vi "stereo_cam_aquisition.vi"() -> ()   [LabVIEW 2015]
uses:
  <vilib>/userdefined/High Color/IMAQdx.ctl
  <vilib>/vision/driver/IMAQdx.llb/IMAQdx Acquisition Mode.ctl
  <vilib>/vision/driver/NI_Vision_Acquisition_Software.lvlib
  <vilib>/Analysis/NI_AALBase.lvlib
panel:
  in  "error in":errorcluster
  in  "stop":bool
  in  "bubnum #2":string
  in  "bubnum #1":string
  out "Absolute Difference in Entropy 2":dbl(graph)
  out "Absolute Difference in Entropy":dbl(graph)
  out "Camera Triggered":bool
  in  "Entropy Threshold":dbl
  out "Camera Image 2":T1(plugin-control)
  out "Buffer #2":u32
  out "Camera Image 1":T1(plugin-control)
  out "Buffer #1":u32
  in  "IMAQdx Session 2":T2
  in  "IMAQdx Session 1":T2
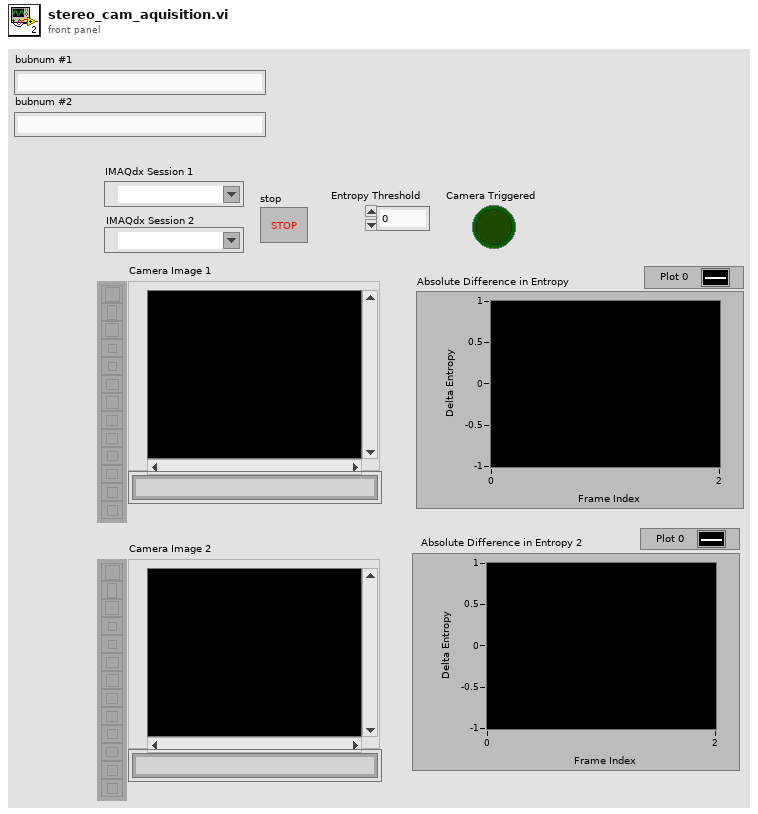
[diagram p1: front panel]
types:
  T1 = typedef "IMAQ Image.ctl" = refnum<image>
  T2 = typedef "IMAQdx.ctl" = refnum<k21>
  T3 = typedef "NI_Vision_Acquisition_Software.lvlib/IMAQdx Acquisition Mode.ctl" = enum32{"One Shot", "Continuous"}
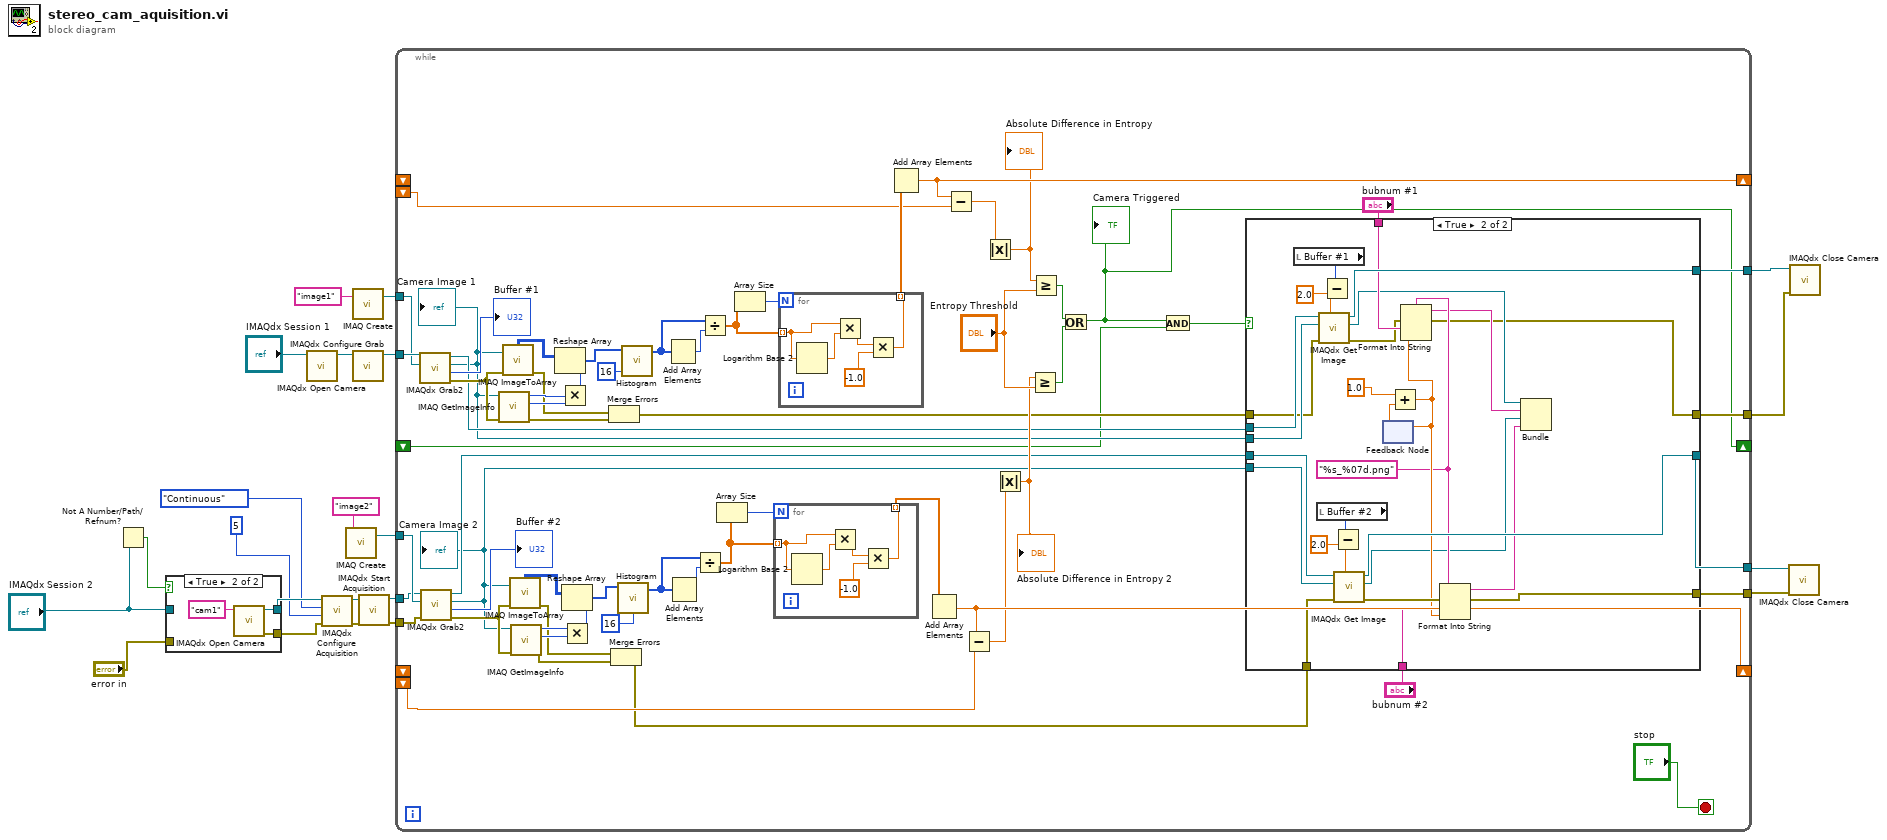
[diagram p0: block diagram]
diagram:
  n1 = Not A Number/Path/Refnum?(number/path/refnum="IMAQdx Session 2") -> (NaN/Path/Refnum?=w6:bool)
  n2 = case shown="True" w6 {
    tunnel: [w24 w27] -> w9
    tunnel: "IMAQdx Session 2" -> [w24 _]
    tunnel: [w23 w26] -> w10
    tunnel: "error in" -> [w23 _]
    frame False {
    }
    frame True {
      n3 = call <vilib>:"IMAQdx Open Camera.vi"("Session In"="cam1") -> ("error out"=w26:errorcluster, "Session Out"=w27:T2)  [unwired: 9 in]
    }
  }
  n4 = call <vilib>:"IMAQdx Open Camera.vi"("Session In"="IMAQdx Session 1") -> ("Session Out"=w22:T2)  [unwired: 9 in, 1 out]
  n5 = call <vilib>:"IMAQdx Configure Acquisition.vi"("error in"=w10, "Number of Buffers"=u32 5, "Continuous?"=IMAQdx_Acquisition_Mode."Continuous", "Session In"=w9) -> ("error out"=w4:errorcluster, "Session Out"=w3:T2)  [unwired: 6 in]
  n6 = call "IMAQ Create"("Image Name"="image2") -> ("New Image"=w18:T1)  [unwired: 4 in, 1 out]
  n7 = call "IMAQ Create"("Image Name"="image1") -> ("New Image"=w16:T1)  [unwired: 4 in, 1 out]
  n8 = call <vilib>:"IMAQdx Configure Grab.vi"("Session In"=w22) -> ("Session Out"=w17:T2)  [unwired: 9 in, 1 out]
  n9 = call <vilib>:"IMAQdx Start Acquisition.vi"("error in"=w4, "Session In"=w3) -> ("error out"=w1:errorcluster, "Session Out"=w2:T2)  [unwired: 8 in]
  n10 = while {
    tunnel: w18 -> [w74]
    tunnel: w17 -> [w73]
    tunnel: w16 -> [w72]
    shift-right: [w70] -> _
    shift-left: _ -> [_]
    shift-left: _ -> [w71]
    shift-right: [w58] -> _
    shift-left: _ -> [_]
    shift-left: _ -> [w55]
    tunnel: [w39] -> w12
    tunnel: [w38] -> w14
    tunnel: [w37] -> w15
    tunnel: [w36] -> w13
    shift-right: [w31] -> _
    shift-left: _ -> [w30]
    tunnel: w2 -> [w29]
    tunnel: w1 -> [w28]
    stop <- "stop" stop-if-true
    n11 = call <vilib>:"IMAQdx Grab2.vi"("Image In"=w72, "Session In"=w73) -> ("error out"=w89:errorcluster, "Buffer Number Out"=→"Buffer #1":u32, "Image Out"=w47:T1, "Session Out"=w48:T2)  [unwired: 6 in]
    "Camera Image 1" <- w47
    n12 = call <vilib>:"IMAQdx Grab2.vi"("error in"=w28, "Image In"=w74, "Session In"=w29) -> ("error out"=w86:errorcluster, "Buffer Number Out"=→"Buffer #2":u32, "Image Out"=w46:T1, "Session Out"=w49:T2)  [unwired: 5 in]
    "Camera Image 2" <- w46
    n13 = call "IMAQ GetImageInfo"("error in (no error)"=w89, "Image"=w47) -> ("error out"=w42:errorcluster, "Y Resolution"=w81:i32, "X Resolution"=w82:i32)  [unwired: 2 in, 5 out]
    n14 = call "IMAQ ImageToArray"("error in (no error)"=w89, "Image"=w47) -> ("error out"=w43:errorcluster, "Image Pixels (U8)"=w80:u8[][])  [unwired: 2 in, 3 out]
    n15 = call "IMAQ ImageToArray"("error in (no error)"=w86, "Image"=w46) -> ("error out"=w45:errorcluster, "Image Pixels (U8)"=w59:u8[][])  [unwired: 2 in, 3 out]
    n16 = call "IMAQ GetImageInfo"("error in (no error)"=w86, "Image"=w46) -> ("error out"=w44:errorcluster, "Y Resolution"=w60:i32, "X Resolution"=w61:i32)  [unwired: 2 in, 5 out]
    n17 = Multiply(x=w82, y=w81) -> (x*y=w83:i32)
    n18 = Reshape Array(w80, w83) -> (w78:u8[])
    n19 = Multiply(x=w61, y=w60) -> (x*y=w64:i32)
    n20 = Reshape Array(w59, w64) -> (w66:u8[])
    n21 = Merge Errors(w43, w42) -> (w41:errorcluster)
    n22 = Merge Errors(w45, w44) -> (w40:errorcluster)
    n23 = call <vilib>:"Histogram.vi"("intervals"=16, "X"=w66) -> ("Histogram: h(x)"=w62:i32[])  [unwired: 6 in, 3 out]
    n24 = call <vilib>:"Histogram.vi"("intervals"=16, "X"=w78) -> ("Histogram: h(x)"=w85:i32[])  [unwired: 6 in, 3 out]
    n25 = Add Array Elements(numeric array=w85) -> (sum=w84:i32)
    n26 = Add Array Elements(numeric array=w62) -> (sum=w63:i32)
    n27 = Divide(x=w62, y=w63) -> (x/y=w68:dbl[])
    n28 = Divide(x=w85, y=w84) -> (x/y=w76:dbl[])
    n29 = Array Size(array=w68) -> (size(s)=w67:i32)
    n30 = Array Size(array=w76) -> (size(s)=w77:i32)
    n31 = for {
      N: w67 -> [_]
      tunnel: w68 -> [w123] mode=indexing
      tunnel: [w122] -> w57 mode=indexing
      n32 = Logarithm Base 2(1:w123) -> (0:w124:dbl)
      n33 = Multiply(x=w123, y=w124) -> (x*y=w125:dbl)
      n34 = Multiply(x=w125, y=-1.0) -> (x*y=w122:dbl)
    }
    n35 = for {
      N: w77 -> [_]
      tunnel: w76 -> [w128] mode=indexing
      tunnel: [w127] -> w75 mode=indexing
      n36 = Logarithm Base 2(1:w128) -> (0:w129:dbl)
      n37 = Multiply(x=w128, y=w129) -> (x*y=w130:dbl)
      n38 = Multiply(x=w130, y=-1.0) -> (x*y=w127:dbl)
    }
    n39 = Add Array Elements(numeric array=w75) -> (sum=w70:dbl)
    n40 = Add Array Elements(numeric array=w57) -> (sum=w58:dbl)
    n41 = Subtract(x=w70, y=w71) -> (x-y=w69:dbl)
    n42 = Subtract(x=w58, y=w55) -> (x-y=w56:dbl)
    n43 = Absolute Value(x=w69) -> (abs(x)=w51:dbl)
    "Absolute Difference in Entropy" <- w51
    n44 = Absolute Value(x=w56) -> (abs(x)=w50:dbl)
    "Absolute Difference in Entropy 2" <- w50
    n45 = Greater Or Equal?(x=w50, y="Entropy Threshold") -> (x >= y?=w52:bool)
    n46 = Greater Or Equal?(x=w51, y="Entropy Threshold") -> (x >= y?=w53:bool)
    n47 = Or(x=w53, y=w52) -> (x .or. y?=w31:bool)
    "Camera Triggered" <- w31
    n48 = And(x=w31, y=w30) -> (x .and. y?=w32:bool)
    n49 = case shown="True" w32 {
      tunnel: w49 -> [w90 w119]
      tunnel: w48 -> [w92 w121]
      tunnel: w47 -> [_ w120]
      tunnel: w46 -> [_ w118]
      tunnel: w41 -> [w91 w117]
      tunnel: w40 -> [w93 w116]
      tunnel: [w93 w94] -> w39
      tunnel: [w92 w114] -> w37
      tunnel: [w91 w95] -> w38
      tunnel: [w90 w115] -> w36
      tunnel: "bubnum #2" -> [_ w113]
      tunnel: "bubnum #1" -> [_ w112]
      frame False {
      }
      frame True {
        w101 = "%s_%07d.png"
        n50 = local read "Buffer #1"() -> (w111:u32)
        n51 = local read "Buffer #2"() -> (w107:u32)
        n52 = Subtract(x=w111, y=2.0) -> (x-y=w110:dbl)
        n53 = call <vilib>:"IMAQdx Get Image.vi"("Buffer Number Mode (Next)"=w110, "error in"=w117, "Image In"=w120, "Session In"=w121) -> ("error out"=w104:errorcluster, "Image Out"=w99:T1, "Session Out"=w114:T2)  [unwired: 1 in, 4 out]
        n54 = Subtract(x=w107, y=2.0) -> (x-y=w108:dbl)
        n55 = call <vilib>:"IMAQdx Get Image.vi"("Buffer Number Mode (Next)"=w108, "error in"=w116, "Image In"=w118, "Session In"=w119) -> ("error out"=w105:errorcluster, "Image Out"=w98:T1, "Session Out"=w115:T2)  [unwired: 1 in, 4 out]
        n56 = feedback #1() -> (w103:dbl)  [unwired: 1 in]
        n57 = Add(x=1.0, y=w103) -> (x+y=w102:dbl)
        n58 = feedback-in #1(w102) -> ()
        n59 = Format Into String(format string=w101, error in=w104, w112, w102) -> (resulting string=w97:string, error out=w95:errorcluster)  [unwired: 1 in]
        n60 = Format Into String(format string=w101, error in=w105, w113, w102) -> (resulting string=w96:string, error out=w94:errorcluster)  [unwired: 1 in]
        n61 = Bundle("Image Out"=w99, w97, "Image Out"=w98, w96) -> ()  [unwired: 1 in, 1 out]
      }
    }
  }
  n62 = call <vilib>:"IMAQdx Close Camera.vi"("error in"=w12, "Session In"=w13) -> ()  [unwired: 9 in, 1 out]
  n63 = call <vilib>:"IMAQdx Close Camera.vi"("error in"=w14, "Session In"=w15) -> ()  [unwired: 9 in, 1 out]
